vi "PY_image_stat.vi"() -> ()   [LabVIEW 2010]
uses:
  <userlib>/labpython/PYTHON Set Float Vector__ogtk.vi
panel:
  in  "stop":bool
  out "Exec Time (ms)":u32
  out "Std. Dev.":dbl
  out "Mediane":dbl
  out "Moyenne":dbl
  in  "array":dbl[](array[numeric])=[11.0, 12.0, 13.0, 14.0] format="%.2f"
  out "error out":errorcluster
  in  "error in (no error)":errorcluster
  in  "script":string="def listType1D(listToCheck=[]):\n    # check if empty list\n    if listToCheck == []:\n        return None\n    else:\n        #initialize sameTypes to TRUE\n        sameTypes = 1\n        #initialize listType to type of 1st element\n        listType = type(listToCheck[0])\n        #iterate thru list checking each elements type\n        for listElement in listToCheck:\n            # if same type then loop again\n            if type(listElement) == listType:\n                pass\n            #if not then break loop and return None\n            else:\n                sameTypes = 0\n                listType = None\n                break\n        # if loop completes then return the listType\n        return listType\n\nfloattype =  listType1D(floatmatrix)\nstringtype = listType1D(stringlist)"
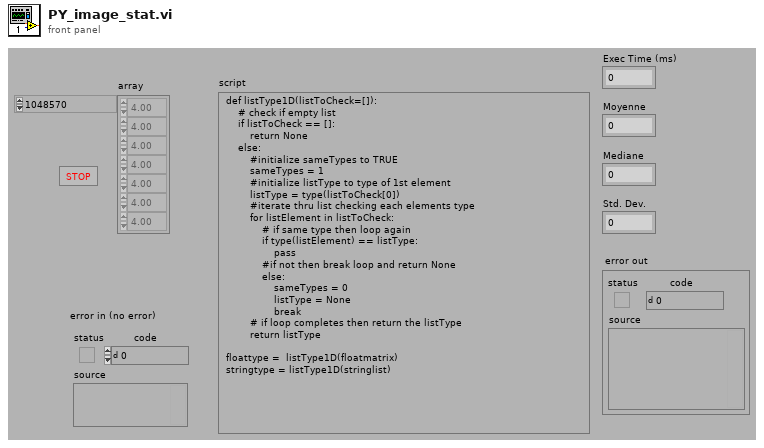
[diagram p1: front panel]
types:
  T1 = typedef "Python Session Refnum__ogtk.ctl" = refnum<k1>
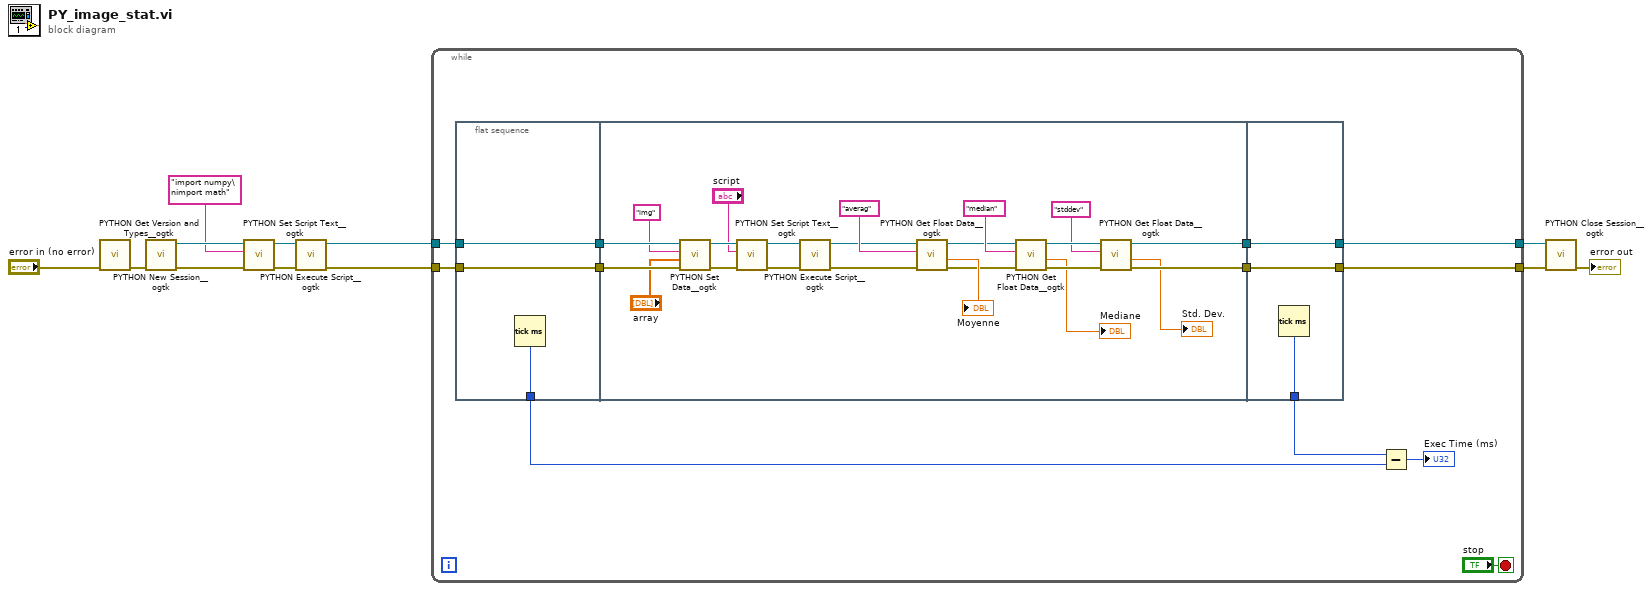
[diagram p0: block diagram]
diagram:
  n1 = call <userlib>:"PYTHON Get Version and Types__ogtk.vi"("error in (no error)"="error in (no error)") -> ("error out"=w12:errorcluster)  [unwired: 4 in, 2 out]
  n2 = call <userlib>:"PYTHON New Session__ogtk.vi"("error in (no error)"=w12) -> ("error out"=w6:errorcluster, "Python Session"=w7:T1)  [unwired: 5 in]
  n3 = call <userlib>:"PYTHON Set Script Text__ogtk.vi"("error in (no error)"=w6, "script text"="import numpy\nimport math", "Python Session in"=w7) -> ("error out"=w3:errorcluster, "Python Session out"=w4:T1)  [unwired: 3 in]
  n4 = call <userlib>:"PYTHON Execute Script__ogtk.vi"("error in (no error)"=w3, "Python Session in"=w4) -> ("error out"=w1:errorcluster, "Python Session out"=w2:T1)  [unwired: 4 in]
  n5 = while {
    tunnel: [w20] -> w9
    tunnel: [w19] -> w8
    tunnel: w2 -> [w15]
    tunnel: w1 -> [w14]
    stop <- "stop" stop-if-true
    n6 = flat-sequence {
      tunnel: w14 -> [w26]
      tunnel: w15 -> [w27]
      tunnel: [w27] -> w24
      tunnel: [w26] -> w23
      tunnel: [w25] -> w17
      tunnel: w24 -> [w50]
      tunnel: w23 -> [w49]
      tunnel: [w48] -> w22
      tunnel: [w47] -> w21
      tunnel: [w52] -> w19
      tunnel: [w53] -> w20
      tunnel: w22 -> [w53]
      tunnel: w21 -> [w52]
      tunnel: [w51] -> w18
      frame #0 {
        n7 = Tick Count (ms)() -> (millisecond timer value=w25:u32)
      }
      frame #1 {
        n8 = call-poly <userlib>:"PYTHON Set Data__ogtk.vi"("error in (no error)"=w49, "value"="array", "variable name"="img", "Python Session in"=w50) -> ("error out"=w41:errorcluster, "Python Session out"=w45:T1)  [unwired: 2 in]
        n9 = call <userlib>:"PYTHON Set Script Text__ogtk.vi"("error in (no error)"=w41, "script text"="script", "Python Session in"=w45) -> ("error out"=w42:errorcluster, "Python Session out"=w43:T1)  [unwired: 3 in]
        n10 = call <userlib>:"PYTHON Execute Script__ogtk.vi"("error in (no error)"=w42, "Python Session in"=w43) -> ("error out"=w31:errorcluster, "Python Session out"=w32:T1)  [unwired: 4 in]
        n11 = call <userlib>:"PYTHON Get Float Data__ogtk.vi"("error in (no error)"=w31, "variable name"="averag", "Python Session in"=w32) -> ("error out"=w28:errorcluster, "value"=→"Moyenne":dbl, "Python Session out"=w30:T1)  [unwired: 2 in]
        n12 = call <userlib>:"PYTHON Get Float Data__ogtk.vi"("error in (no error)"=w28, "variable name"="median", "Python Session in"=w30) -> ("error out"=w38:errorcluster, "value"=→"Mediane":dbl, "Python Session out"=w39:T1)  [unwired: 2 in]
        n13 = call <userlib>:"PYTHON Get Float Data__ogtk.vi"("error in (no error)"=w38, "variable name"="stddev", "Python Session in"=w39) -> ("error out"=w47:errorcluster, "value"=→"Std. Dev.":dbl, "Python Session out"=w48:T1)  [unwired: 2 in]
      }
      frame #2 {
        n14 = Tick Count (ms)() -> (millisecond timer value=w51:u32)
      }
    }
    n15 = Subtract(x=w18, y=w17) -> (x-y=→"Exec Time (ms)":u32)
  }
  n16 = call <userlib>:"PYTHON Close Session__ogtk.vi"("error in (no error)"=w8, "Python Session in"=w9) -> ("error out"=→"error out":errorcluster)  [unwired: 5 in]
